vi "Do.vi"(8 "error in (no error)":errorcluster, 10 "Actor in":refnum<class "Actor.lvclass">, 11 "Create Room Service Request Msg":refnum<class "Create Room Service Request Msg.lvclass">) -> (0 "error out":errorcluster, 2 "Actor out":refnum<class "Actor.lvclass">)   [LabVIEW 2023, in "Room Service Manager Model.lvlib" / "Create Room Service Request Msg.lvclass"]
doc: "This VI delivers the message to the actor by calling the appropriate method(s) on the actor."
uses:
  Create Room Service Request Msg.lvclass
  Create Room Service Request Msg.lvclass/Create Room Service Request Msg.ctl
  34700b1e-4b1b-4205-ab4b-28631ba2a4c6.vi
  Room Service Manager Model/Room Service Manager Model.lvclass
  Room Service Manager UI/Room Service Manager UI Messages/Create Room Service Request Msg/Create Room Service Request Msg.lvclass
  C:/Users/bhaghyaraj/Trainings/NI Actor Framework/SDLC/Room Service Manager UI/Room Service Manager UI Messages/Create Room Service Request Msg/Create Room Service Request Msg.lvclass
  C:/Program Files/National Instruments/LabVIEW 2023/vi.lib/ActorFramework/Message/Message.lvclass
  C:/Users/bhaghyaraj/Trainings/NI Actor Framework/SDLC/Room Service Manager Model/Room Service Manager Model Messages/Create Room Service Request Msg/Create Room Service Request Msg.lvclass
  <vilib>/ActorFramework/Actor/Actor.lvclass
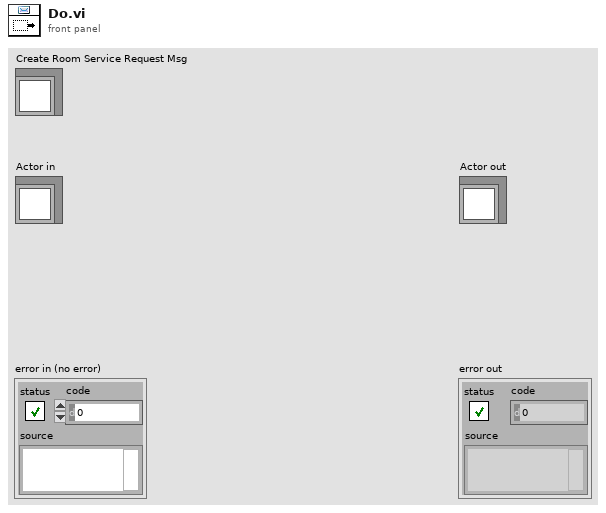
[diagram p1: front panel]
types:
  T1 = cluster{"Room Service":refnum<class "Room Service Base.lvclass">}
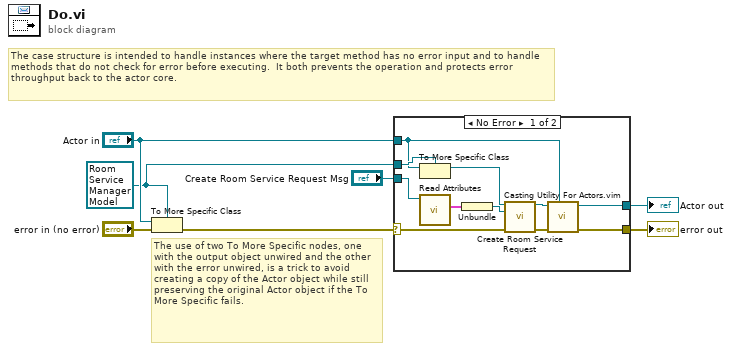
[diagram p0: block diagram]
diagram:
  w2 = refnum<class "Room Service Manager Model.lvclass"> refnum ("Actor in")
  # "The use of two To More Specific nodes, one with the output object unwired and the other with the error unwired, is a trick to avoid creating a copy of the Actor object while still preserving the original Actor object if the To More Specific fails."
  # "The case structure is intended to handle instances where the target method has no error input and to handle methods that do not check for error before executing.  It both prevents the operation and protects error throughput back to the actor core."
  n1 = To More Specific Class(target class=w2, reference="Actor in", error in="error in (no error)") -> (error out=w6:errorcluster)  [unwired: 1 out]
  n2 = case shown="No Error" w6 {
    selector: w6 -> [w18 w20]
    tunnel: [w10 w20] -> w5
    tunnel: [w9 w19] -> w4
    tunnel: "Actor in" -> [w13 w19]
    tunnel: w2 -> [w14 _]
    tunnel: "Create Room Service Request Msg" -> [w15 _]
    frame No Error {
      n3 = To More Specific Class(target class=w14, reference=w13) -> (specific class reference=w17:refnum<class "Room Service Manager Model.lvclass">)  [unwired: 1 in, 1 out]
      n4 = call "Read Attributes.vi"("Create Room Service Request Msg"=w15) -> ("Payload"=w16:T1)  [unwired: 10 in]
      n5 = Unbundle(w16) -> ("Room Service"=w8:refnum<class "Room Service Base.lvclass">)
      n6 = call-dynamic "Create Room Service Request.vi"("Room Service Manager Model in"=w17, "Room Service"=w8, "error in (no error)"=w18) -> ("Room Service Manager Model out"=w12:refnum<class "Room Service Manager Model.lvclass">, "error out"=w11:errorcluster)  [unwired: 11 in]
      n7 = call "Casting Utility For Actors.vim"("type"=w13, "error in (no error)"=w11, "Actor in"=w12) -> ("error out"=w10:errorcluster, "Actor out"=w9:refnum<class "Actor.lvclass">)  [unwired: 7 in]
    }
    frame Error {
      # "If type check fails, pass the original object out again."
    }
  }
  "error out" <- w5
  "Actor out" <- w4
